vi "Multi Cycle Reset.vi"(1 "reset (strobe)":bool) -> (4 "reset (fanout)":bool)   [LabVIEW 2020, in "GettingStarted_Common_148X_FPGA.lvlib"]
uses:
  GettingStarted_Common_148X_FPGA.lvlib
  <instrlib>/_niInstr/Basic Elements/v1/FPGA/Private/Count Up U16.vi
  <instrlib>/_niInstr/Basic Elements/v1/FPGA/niInstr Basic Elements v1 FPGA.lvlib
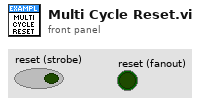
[diagram p1: front panel]
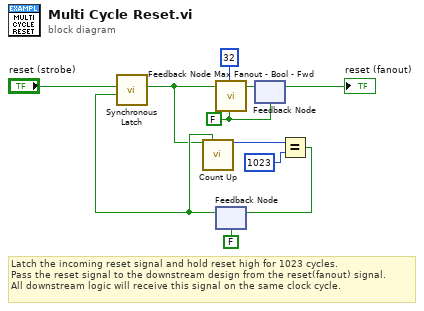
[diagram p0: block diagram]
diagram:
  w1 = FALSE
  # "Latch the incoming reset signal and hold reset high for 1023 cycles.\nPass the reset signal to the downstream design from the reset(fanout) signal.\nAll downstream logic will receive this signal on the same clock cycle."
  n1 = feedback #1(FALSE) -> (w8:bool)
  n2 = call <instrlib>:"Synchronous Latch.vi"("clear"=w8, "set"="reset (strobe)") -> ("out"=w3:bool)  [unwired: 9 in]
  n3 = call-poly <instrlib>:"Count Up.vi"("increment"=w3, "reset"=w8) -> ("count out"=w11:u16)  [unwired: 13 in]
  n4 = call <instrlib>:"Feedback Node Max Fanout - Bool - Fwd.vi"("cDataIn"=w3, "kMaxFanout"=u8 32, "kInitialValue"=w1) -> ("cDataOut"=w4:bool)  [unwired: 24 in]
  n5 = feedback-in #2(w4) -> ()
  n6 = feedback #2(w1) -> (→"reset (fanout)":bool)
  n7 = Equal?(x=w11, y=u16 1023) -> (x = y?=w9:bool)
  n8 = feedback-in #1(w9) -> ()
